vi "Get Limit Test Values.vi"(0 "VISA resource name":refnum<visa-resource-name>, 5 "Function":u16(ring) items=["Voltage: DC", "Voltage: AC", "Current: DC", "Current: AC", "2W Resistance", "4W Resistance", "Diode", "Capacitance", "Temperature", "Continuity", "Frequency", "Period", "Ratio", "Digitize Voltage", "Digitize Current"], 7 "Limit Test Number":u16=1 min=1 max=2 step=1, 11 "error in (no error)":errorcluster) -> (4 "VISA resource name out":refnum<visa-resource-name>, 6 "Lower Limit":dbl, 8 "Upperr Limit":dbl, 15 "error out":errorcluster)   [LabVIEW 2025, in "Keithley DMM7510.lvlib"]
doc: "This VI queries the lower and upper limit values for limit tests."
uses:
  Keithley DMM7510.lvlib
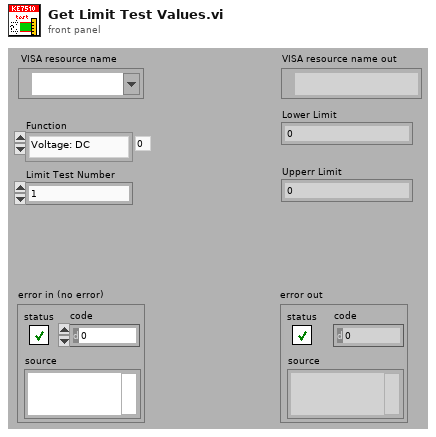
[diagram p1: front panel]
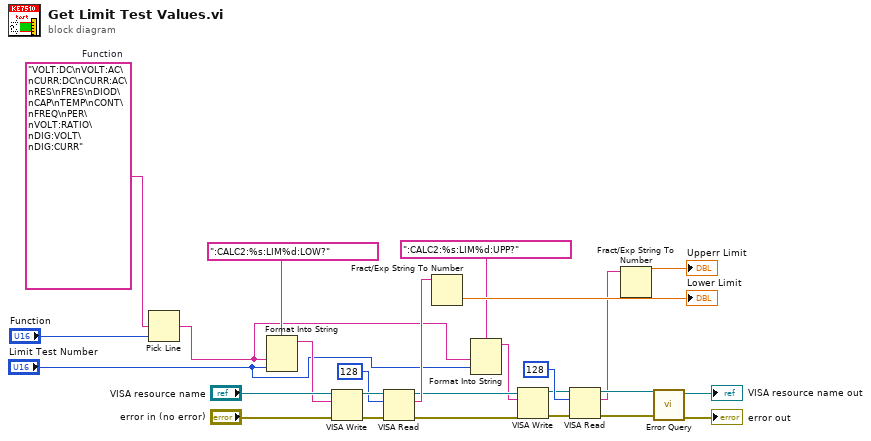
[diagram p0: block diagram]
diagram:
  w15 = "VOLT:DC\nVOLT:AC\nCURR:DC\nCURR:AC\nRES\nFRES\nDIOD\nCAP\nTEMP\nCONT\nFREQ\nPER\nVOLT:RATIO\nDIG:VOLT\nDIG:CURR"  # Function
  n1 = Pick Line(multi-line string=w15, line index="Function") -> (output string=w12:string)  [unwired: 1 out]
  n2 = Format Into String(format string=":CALC2:%s:LIM%d:LOW?", w12, "Limit Test Number") -> (resulting string=w22:string)  [unwired: 2 in, 1 out]
  n3 = VISA Write(VISA resource name="VISA resource name", write buffer=w22, error in (no error)="error in (no error)") -> (VISA resource name out=w20:refnum<visa-resource-name>, error out=w21:errorcluster)  [unwired: 1 out]
  n4 = VISA Read(VISA resource name=w20, byte count=u32 128, error in (no error)=w21) -> (VISA resource name out=w9:refnum<visa-resource-name>, read buffer=w18:string, error out=w8:errorcluster)  [unwired: 1 out]
  n5 = Fract/Exp String To Number(string=w18) -> (number=→"Lower Limit":dbl)  [unwired: 3 in, 1 out]
  n6 = Format Into String(format string=":CALC2:%s:LIM%d:UPP?", w12, "Limit Test Number") -> (resulting string=w7:string)  [unwired: 2 in, 1 out]
  n7 = VISA Write(VISA resource name=w9, write buffer=w7, error in (no error)=w8) -> (VISA resource name out=w6:refnum<visa-resource-name>, error out=w5:errorcluster)  [unwired: 1 out]
  n8 = VISA Read(VISA resource name=w6, byte count=u32 128, error in (no error)=w5) -> (VISA resource name out=w4:refnum<visa-resource-name>, read buffer=w1:string, error out=w3:errorcluster)  [unwired: 1 out]
  n9 = Fract/Exp String To Number(string=w1) -> (number=→"Upperr Limit":dbl)  [unwired: 3 in, 1 out]
  n10 = call "Error Query.vi"("error in (no error)"=w3, "VISA resource name"=w4) -> ("error out"=→"error out":errorcluster, "VISA resource name out"=→"VISA resource name out":refnum<visa-resource-name>)  [unwired: 8 out]
